vi "Untitled 2.vi"() -> ()   [LabVIEW 2026]
uses:
  <vilib>/Wovalab/Utilities/Helper Loop Periodic Timing/Late Execution Mode--enum.ctl
  <vilib>/Wovalab/Utilities/Helper Loop Periodic Timing/Helper Loop Periodic Timing.lvclass/Helper Loop Periodic Timing.ctl
  <vilib>/Wovalab/Utilities/Helper Loop Periodic Timing/Stop Helper Loop Internal.vi
  <vilib>/Wovalab/Utilities/Helper Loop Periodic Timing/U32 Max Value--constant.vi
  <vilib>/Wovalab/Utilities/Helper Loop Periodic Timing/Update Last Execution Time.vi
  <vilib>/Wovalab/Utilities/Helper Loop Periodic Timing/Loops Events AE.vi
  <vilib>/Wovalab/Utilities/Helper Loop Periodic Timing/Notify Monitoring Window.vi
  <vilib>/Wovalab/Utilities/Helper Loop Periodic Timing/Monitoring--global.vi
  <vilib>/Wovalab/Utilities/Helper Loop Periodic Timing/Helper Loop Periodic Timing.lvclass
  User32.dll
panel:
  out "element 2":i32
  out "element":i32
  out "x != 0? 2":bool
  out "x != 0?":bool
  out "seconds since 1Jan1904":timestamp
  in  "Exit":bool
  in  "Stop":bool
  in  "Start":bool
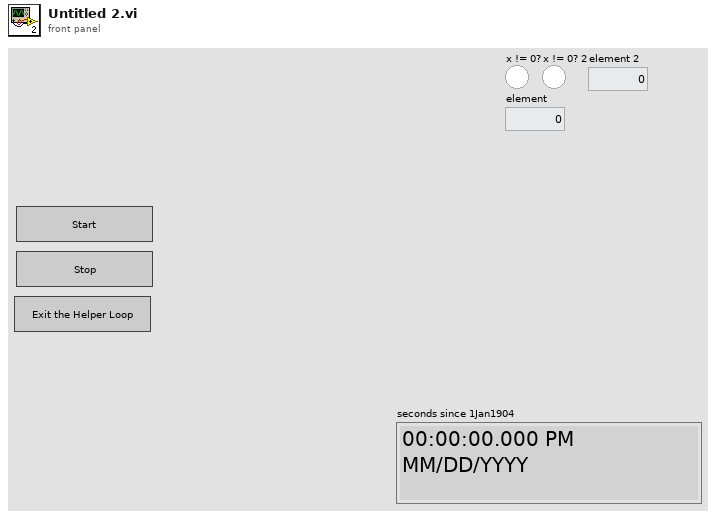
[diagram p1: front panel]
types:
  T1 = typedef "Wovalab_lib_Utilities.lvlib/Helper Loop Periodic Timing.lvclass/Late Execution Mode--enum.ctl" = enum16{"No change", "Process missed periods ignoring original phase", "Process missed periods maintaining original phase"}
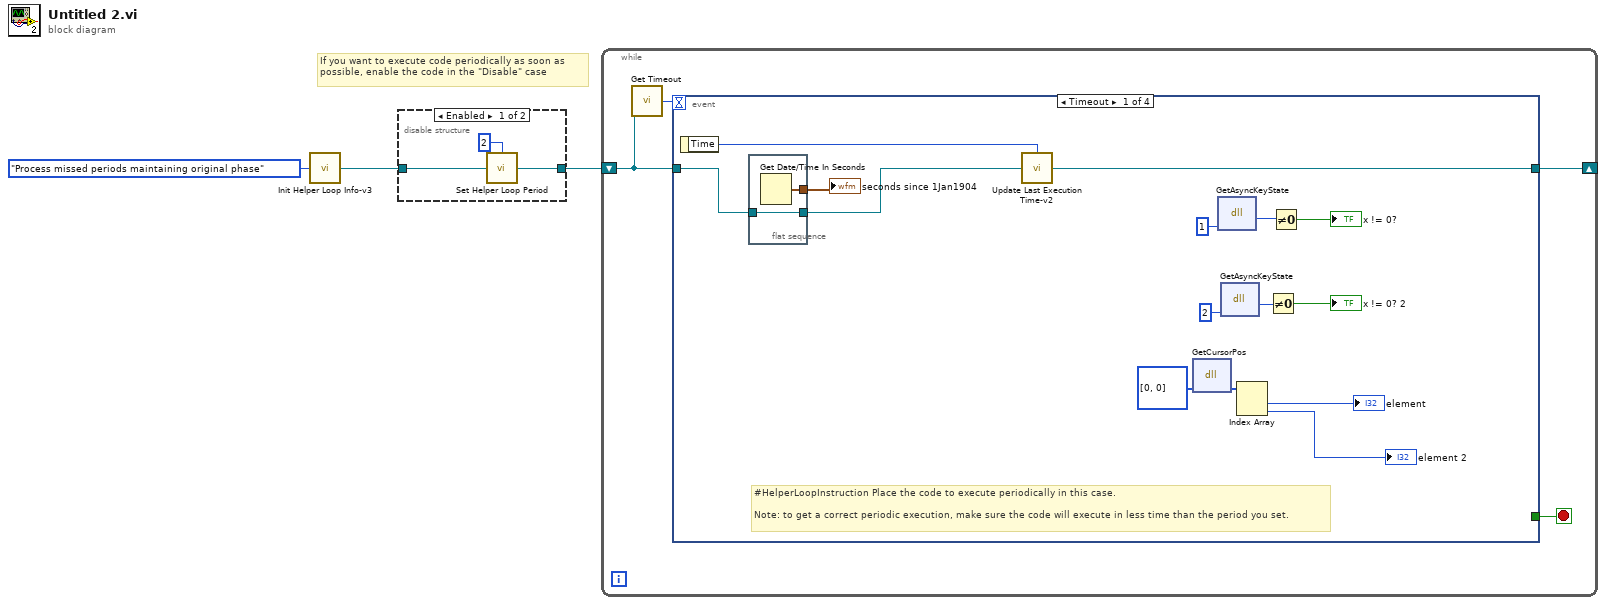
[diagram p0: block diagram]
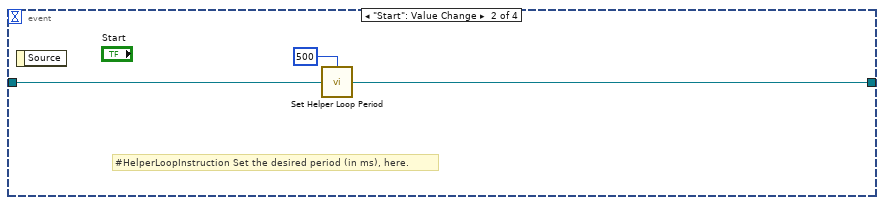
[diagram p3: hidden frame]
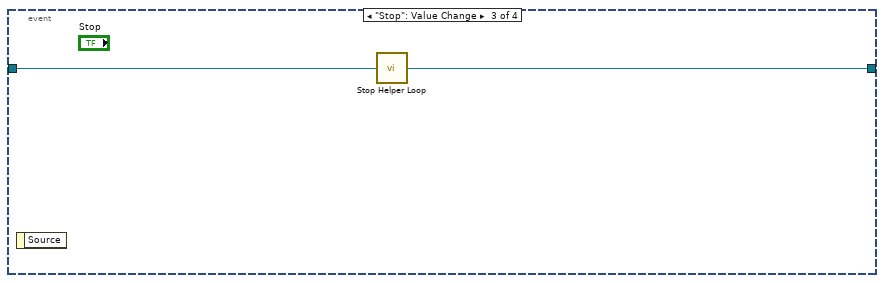
[diagram p4: hidden frame]
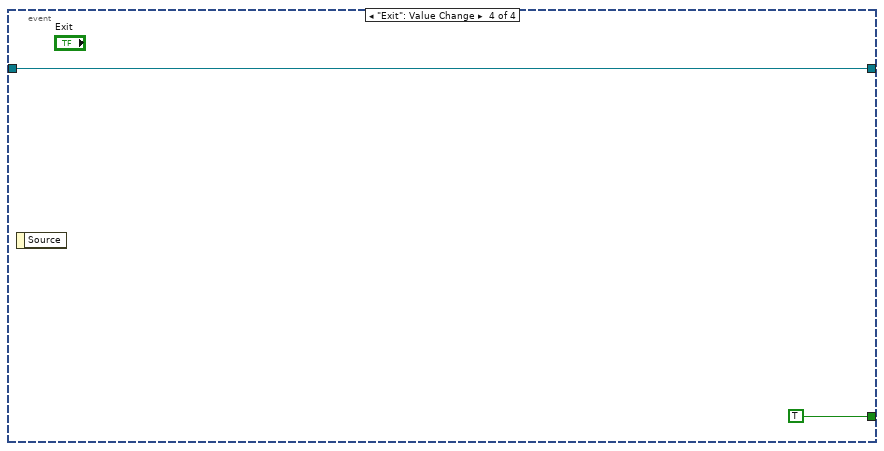
[diagram p5: hidden frame]
diagram:
  # "If you want to execute code periodically as soon as possible, enable the code in the \"Disable\" case"
  n1 = call <vilib>:"Init Helper Loop Info-v3.vi"("Late Execution Mode (Process missed periods ignoring original phase)"=Late_Execution_Mode--enum."Process missed periods maintaining original phase") -> ("Helper Loop Periodic Timing"=w2:refnum<class "Helper Loop Periodic Timing.lvclass">)  [unwired: 1 in]
  n2 = disable-structure shown="Enabled" {
    disable-tunnel: w2 -> [w6 w7]
    disable-tunnel: [w5 w7] -> w3
    frame Enabled {
      n3 = call <vilib>:"Set Helper Loop Period.vi"("Period (ms)"=2, "Helper Loop Periodic Timing in"=w6) -> ("Helper Loop Periodic Timing out"=w5:refnum<class "Helper Loop Periodic Timing.lvclass">)  [unwired: 13 in]
    }
    frame Disabled {
    }
  }
  n4 = while {
    shift-right: [w9] -> _
    shift-left: w3 -> [w10]
    stop <- w8 stop-if-true
    n5 = call <vilib>:"Get Timeout.vi"("Helper Loop Periodic Timing"=w10) -> ("Timeout (ms)"=w11:i32)  [unwired: 12 in, 2 out]
    n6 = event shown="[0] Timeout" {
      selector: _ -> [_ _ _ _]
      dyn-events: _ -> [_ _ _ _]
      timeout: w11 -> [_ _ _ _]
      tunnel: w10 -> [w25 w31 w33 w35]
      tunnel: [w22 w30 w32 w35] -> w9
      tunnel: [_ _ _ TRUE] -> w8
      event Timeout {
        # "#HelperLoopInstruction Place the code to execute periodically in this case.\n\nNote: to get a correct periodic execution, make sure the code will execute in less time than the period you set."
        n7 = event-data() -> ("Time"=w26:u32)  [unwired: 1 in]
        n8 = flat-sequence {
          tunnel: w25 -> [w28]
          tunnel: [w28] -> w24
          tunnel: [w27] -> w23
          frame #0 {
            n9 = Get Date/Time In Seconds() -> (seconds since 1Jan1904=w27:timestamp)
          }
        }
        n10 = call <vilib>:"Update Last Execution Time-v2.vi"("Time"=w26, "Helper Loop Periodic Timing in"=w24) -> ("Helper Loop Periodic Timing out"=w22:refnum<class "Helper Loop Periodic Timing.lvclass">)  [unwired: 12 in, 1 out]
        n11 = dll-call lib="User32.dll" fn="GetCursorPos"("Position"=i32[] [0, 0]) -> ("Position"=w20:i32[])  [unwired: 4 in, 2 out]
        n12 = dll-call lib="User32.dll" fn="GetAsyncKeyState" label="Left Button Click"("vKey"=i16 1) -> ("return type"=w17:i16)  [unwired: 4 in, 2 out]
        n13 = dll-call lib="User32.dll" fn="GetAsyncKeyState" label="Right Button Click"("vKey"=i16 2) -> ("return type"=w16:i16)  [unwired: 4 in, 2 out]
        n14 = Index Array(array=w20) -> (element #1=→"element":i32, element #2=→"element 2":i32)  [unwired: 2 in]
        n15 = Not Equal To 0?(x=w16) -> (x != 0?=→"x != 0? 2":bool)
        n16 = Not Equal To 0?(x=w17) -> (x != 0?=→"x != 0?":bool)
        "seconds since 1Jan1904" <- w23
      }
      event "Start": Value Change {
        # "#HelperLoopInstruction Set the desired period (in ms), here."
        n17 = event-data() -> ()  [unwired: 1 in, 1 out]
        n18 = call <vilib>:"Set Helper Loop Period.vi"("Period (ms)"=500, "Helper Loop Periodic Timing in"=w31) -> ("Helper Loop Periodic Timing out"=w30:refnum<class "Helper Loop Periodic Timing.lvclass">)  [unwired: 13 in]
      }
      event "Stop": Value Change {
        n19 = event-data() -> ()  [unwired: 1 in, 1 out]
        n20 = call <vilib>:"Stop Helper Loop.vi"("Helper Loop Periodic Timing in"=w33) -> ("Helper Loop Periodic Timing out"=w32:refnum<class "Helper Loop Periodic Timing.lvclass">)
      }
      event "Exit": Value Change {
        n21 = event-data() -> ()  [unwired: 1 in, 1 out]
      }
    }
  }
